vi "CRYCalc Pp value.vi"(0 "Data values in":T1 {"Z data" items=["dB", "Lin"]; "X data" items=["dB", "Lin"]; "Y data" items=["dB", "Lin"]; "Z dB ref" format="%.1f"; "Z axis" items=["Log", "Lin"]; "X dB ref" format="%.1f"; "X axis" items=["Log", "Lin"]; "Y axis" items=["Log", "Lin"]; "Y dB ref" format="%.1f"; "Curve"."z" format="%.2f"; "Curve"."y" format="%.2f"; "Curve"."x" format="%.2f"}, 1 "Step Setup VI No":i32, 5 "USL":dbl, 9 "LSL":dbl, 11 "Statistic Run Number":i32, 12 "Mode xyz":u16, 13 "Work in":u16) -> (4 "Pp value Out":T1 {"Z data" items=["dB", "Lin"]; "X data" items=["dB", "Lin"]; "Y data" items=["dB", "Lin"]; "Z dB ref" format="%.1f"; "Z axis" items=["Log", "Lin"]; "X dB ref" format="%.1f"; "X axis" items=["Log", "Lin"]; "Y axis" items=["Log", "Lin"]; "Y dB ref" format="%.1f"; "Curve"."z" format="%.2f"; "Curve"."y" format="%.2f"; "Curve"."x" format="%.2f"}, 6 "Mean Out":T1 {"Z data" items=["dB", "Lin"]; "X data" items=["dB", "Lin"]; "Y data" items=["dB", "Lin"]; "Z dB ref" format="%.1f"; "Z axis" items=["Log", "Lin"]; "X dB ref" format="%.1f"; "X axis" items=["Log", "Lin"]; "Y axis" items=["Log", "Lin"]; "Y dB ref" format="%.1f"; "Curve"."z" format="%.2f"; "Curve"."y" format="%.2f"; "Curve"."x" format="%.2f"}, 10 "Absolute StanDev Out":T1 {"Z data" items=["dB", "Lin"]; "X data" items=["dB", "Lin"]; "Y data" items=["dB", "Lin"]; "Z dB ref" format="%.1f"; "Z axis" items=["Log", "Lin"]; "X dB ref" format="%.1f"; "X axis" items=["Log", "Lin"]; "Y axis" items=["Log", "Lin"]; "Y dB ref" format="%.1f"; "Curve"."z" format="%.2f"; "Curve"."y" format="%.2f"; "Curve"."x" format="%.2f"})   [LabVIEW 2013]
uses:
  Typedef Control/CRYData Cluster Array.ctl
  Typedef Control/CRYData Cluster.ctl
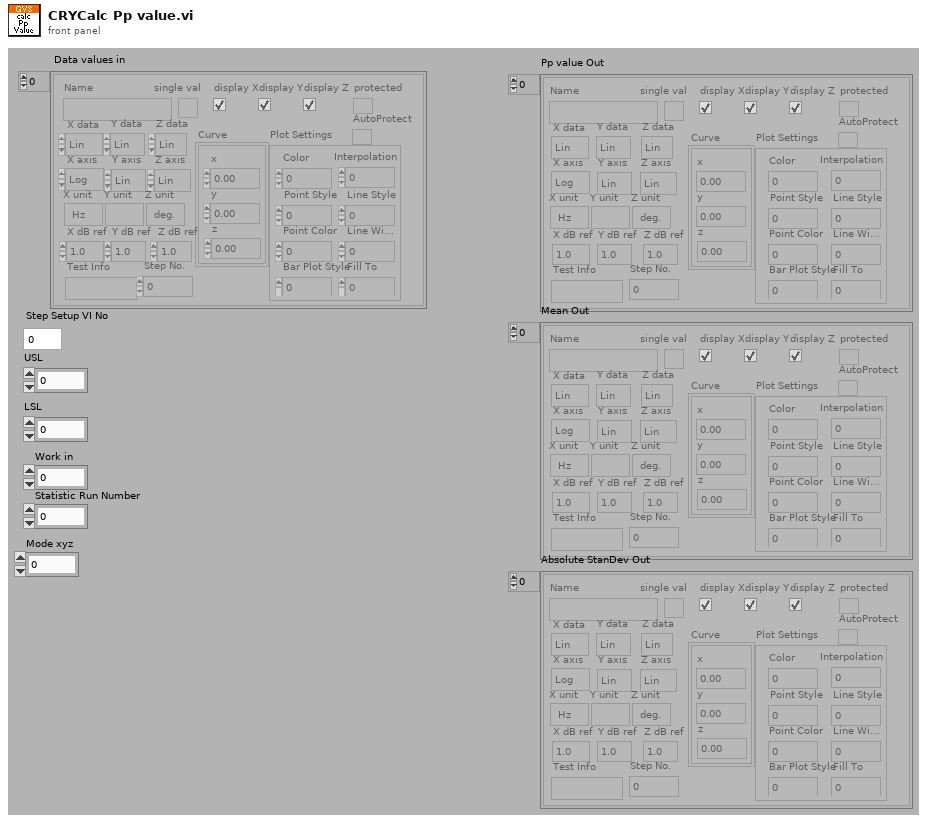
[diagram p1: front panel]
types:
  T1 = typedef "CRYData Cluster Array.ctl" = T2[]
  T2 = typedef "CRYData Cluster.ctl" = cluster{"Name":string, "Curve":cluster{"x":dbl, "y":dbl, "z":dbl}[], "X data":u16, "Y data":u16, "Z data":u16, "X axis":u16, "Y axis":u16, "Z axis":u16, "X unit":string, "Y unit":string, "Z unit":string, "X dB ref":dbl, "Y dB ref":dbl, "Z dB ref":dbl, "single val":bool, "protected":bool, "display X":bool, "display Y":bool, "display Z":bool, "Test Info":string, "Step No.":i32, "Plot Settings":cluster{"Color":u32, "Interpolation":u8, "Point Style":u8, "Line Style":u8, "Point Color":u32, "Line Width":u8, "Bar Plot Style":u8, "Fill To":i16}, "AutoProtect":bool}
  T3 = enum32{"English", "Chinese", "Korean", "Japanese", "Russian", "Chinese traditional"}
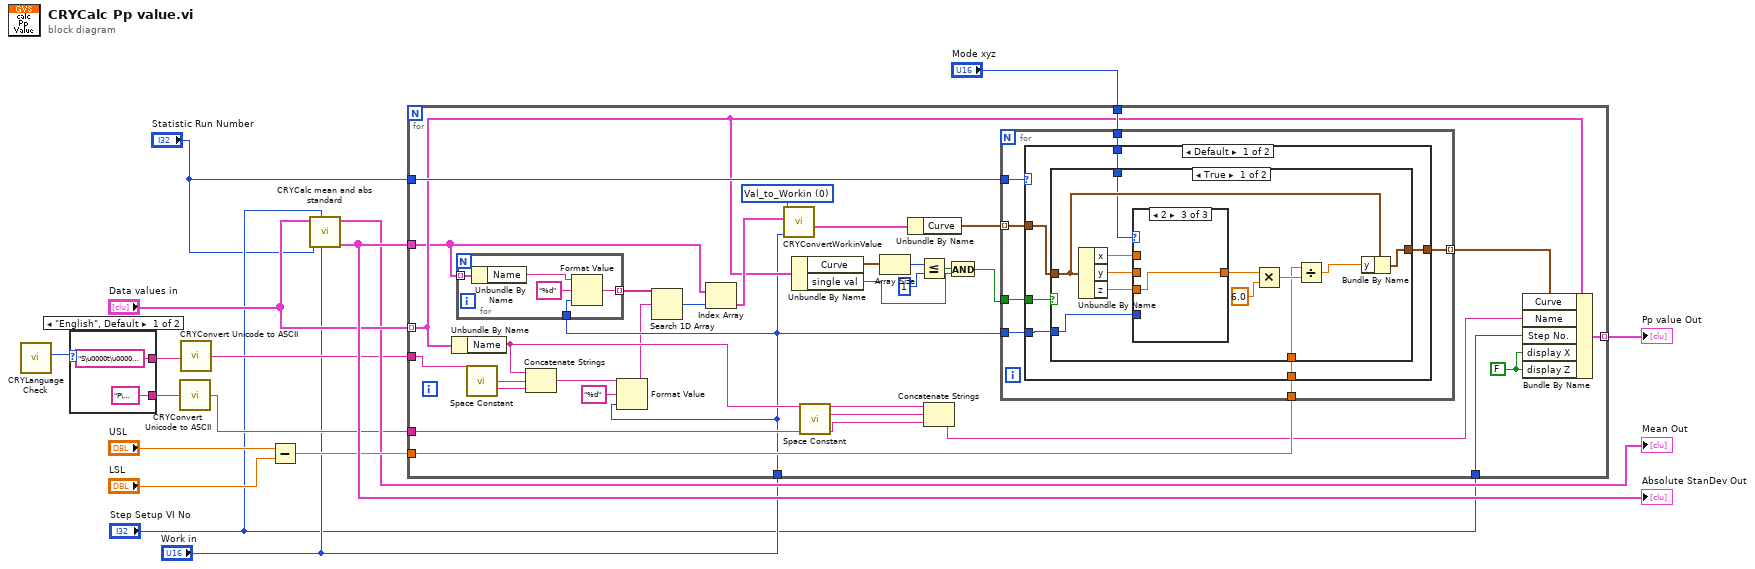
[diagram p0: block diagram]
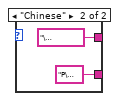
[diagram p2: hidden frame]
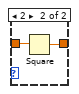
[diagram p5: hidden frame]
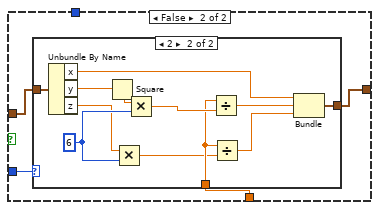
[diagram p6: hidden frame]
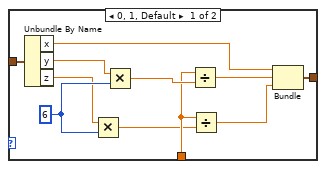
[diagram p7: hidden frame]
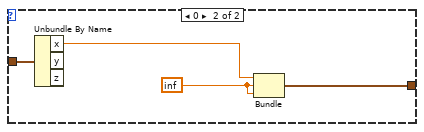
[diagram p8: hidden frame]
diagram:
  n1 = call "CRYLanguage Check.vi"() -> ("Language"=w9:T3)  [unwired: 10 in, 1 out]
  n2 = case shown="\"English\", Default" w9 {
    tunnel: ["S\u0000t\u0000d\u0000 \u0000D\u0000e\u0000v\u0000" ("format string") "\u0007hÆQî]" ("format string")] -> w8
    tunnel: ["P\u0000p\u0000" ("format string") "P\u0000p\u0000" ("format string")] -> w7
    frame "English", Default {
    }
    frame "Chinese" {
    }
  }
  n3 = call "CRYConvert Unicode to ASCII.vi"("Unicode"=w7) -> ("ASCII"=w5:string)  [unwired: 4 in]
  n4 = call "CRYConvert Unicode to ASCII.vi"("Unicode"=w8) -> ("ASCII"=w6:string)  [unwired: 4 in]
  n5 = Subtract(x="USL", y="LSL") -> (x-y=w12:dbl)
  n6 = call "CRYCalc mean and abs standard.vi"("Work in"="Work in", "Step Setup VI No"="Step Setup VI No", "Statistic Run Number"="Statistic Run Number", "Data in"="Data values in") -> ("Absolute StanDev Out"=w14:T1, "Mean Out"=→"Mean Out":T1)  [unwired: 5 in, 1 out]
  "Absolute StanDev Out" <- w14
  n7 = for {
    tunnel: w14 -> [w26]
    tunnel: "Data values in" -> [w27] mode=indexing
    tunnel: w12 -> [w47]
    tunnel: [w37] -> w11 mode=indexing
    tunnel: "Step Setup VI No" -> [w43]
    tunnel: w6 -> [w42]
    tunnel: w5 -> [w41]
    tunnel: "Work in" -> [w22]
    tunnel: "Statistic Run Number" -> [w36]
    tunnel: "Mode xyz" -> [w35]
    w34 = FALSE ("display X")
    w38 = u16 0 items=["Val_to_Workin", "Workin_to_ Val"] ("Type")
    n8 = Unbundle By Name(w27) -> ("Name"=w48:string)
    n9 = for {
      tunnel: w26 -> [w56] mode=indexing
      tunnel: w22 -> [w53]
      tunnel: [w52] -> w25 mode=indexing
      n10 = Unbundle By Name(w56) -> ("Name"=w54:string)
      n11 = Format Value(string ("")=w54, format string="%d", value (0)=w53) -> (output string=w52:string)
    }
    n12 = call <vilib>:"Space Constant.vi"() -> ("String"=w51:string)
    n13 = Concatenate Strings(w48, w51, w42) -> (w23:string)
    n14 = Format Value(string ("")=w23, format string="%d", value (0)=w22) -> (output string=w21:string)
    n15 = Search 1D Array(1D array=w25, element=w21) -> (index of element=w50:i32)  [unwired: 1 in]
    n16 = Index Array(array=w26, index=w50) -> (element=w40:T2)
    n17 = call "CRYConvertWorkinValue.vi"("Work in"=w22, "In"=w40, "Type"=w38) -> ("Out"=w39:T2)  [unwired: 8 in]
    n18 = Unbundle By Name(w27) -> ("Curve"=w33:cluster{"x":dbl, "y":dbl, "z":dbl}[], "single val"=w29:bool)
    n19 = call <vilib>:"Space Constant.vi"() -> ("String"=w49:string)
    n20 = Array Size(array=w33) -> (size(s)=w32:i32)
    n21 = Unbundle By Name(w39) -> ("Curve"=w44:cluster{"x":dbl, "y":dbl, "z":dbl}[])
    n22 = Less Or Equal?(x=w32, y=1) -> (x <= y?=w30:bool)
    n23 = Concatenate Strings(w48, w49, w41) -> (w46:string)
    n24 = And(x=w30, y=w29) -> (x .and. y?=w28:bool)
    n25 = for {
      tunnel: w44 -> [w63] mode=indexing
      tunnel: w47 -> [w62]
      tunnel: [w61] -> w45 mode=indexing
      tunnel: w22 -> [w60]
      tunnel: w36 -> [w59]
      tunnel: w28 -> [w58]
      tunnel: w35 -> [w57]
      n26 = case shown="Default" w59 {
        tunnel: w63 -> [w69 w120]
        tunnel: w62 -> [w68 _]
        tunnel: [w67 w119] -> w61
        tunnel: w60 -> [w66 _]
        tunnel: w58 -> [w65 _]
        tunnel: w57 -> [w64 _]
        frame Default {
          n27 = case shown="True" w65 {
            tunnel: w69 -> [w81 w93]
            tunnel: w68 -> [w73 w92]
            tunnel: [w80 w91] -> w67
            tunnel: w66 -> [w76 w90]
            tunnel: w64 -> [w70 _]
            frame True {
              n28 = Unbundle By Name(w81) -> ("x"=w75:dbl, "y"=w79:dbl, "z"=w74:dbl)
              n29 = case shown="2" w70 {
                tunnel: w79 -> [_ w85 _]
                tunnel: [w82 w84 w89] -> w78
                tunnel: w76 -> [_ w83 _]
                tunnel: w75 -> [w82 _ _]
                tunnel: w74 -> [_ _ w89]
                frame 0, Default {
                }
                frame 1 {
                  n30 = case shown="0, 1, Default" w83 {
                    tunnel: w85 -> [w86 w88]
                    tunnel: [w86 w87] -> w84
                    frame 0, 1, Default {
                    }
                    frame 2 {
                      n31 = Square(x=w88) -> (x^2=w87:dbl)
                    }
                  }
                }
                frame 2 {
                }
              }
              n32 = Multiply(x=w78, y=6.0) -> (x*y=w77:dbl)
              n33 = Divide(x=w73, y=w77) -> (x/y=w71:dbl)
              n34 = Bundle By Name(cluster=w81, "y"=w71) -> (w80:cluster{"x":dbl, "y":dbl, "z":dbl})
            }
            frame False {
              n35 = case shown="2" w90 {
                tunnel: w93 -> [w104 w116]
                tunnel: w92 -> [w101 w113]
                tunnel: [w96 w107] -> w91
                frame 0, 1, Default {
                  w103 = 6 ("standard deviation")
                  n36 = Unbundle By Name(w104) -> ("x"=w98:dbl, "y"=w95:dbl, "z"=w94:dbl)
                  n37 = Multiply(x=w94, y=w103) -> (x*y=w100:dbl)
                  n38 = Multiply(x=w95, y=w103) -> (x*y=w102:dbl)
                  n39 = Divide(x=w101, y=w102) -> (x/y=w99:dbl)
                  n40 = Divide(x=w101, y=w100) -> (x/y=w97:dbl)
                  n41 = Bundle("x"=w98, w99, w97) -> (w96:cluster{"x":dbl, dbl, dbl})  [unwired: 1 in]
                }
                frame 2 {
                  w115 = 6 ("standard deviation")
                  n42 = Unbundle By Name(w116) -> ("x"=w109:dbl, "y"=w111:dbl, "z"=w105:dbl)
                  n43 = Square(x=w111) -> (x^2=w106:dbl)
                  n44 = Multiply(x=w105, y=w115) -> (x*y=w112:dbl)
                  n45 = Multiply(x=w106, y=w115) -> (x*y=w114:dbl)
                  n46 = Divide(x=w113, y=w114) -> (x/y=w110:dbl)
                  n47 = Divide(x=w113, y=w112) -> (x/y=w108:dbl)
                  n48 = Bundle("x"=w109, w110, w108) -> (w107:cluster{"x":dbl, dbl, dbl})  [unwired: 1 in]
                }
              }
            }
          }
        }
        frame 0 {
          w117 = inf
          n49 = Unbundle By Name(w120) -> ("x"=w118:dbl)  [unwired: 2 out]
          n50 = Bundle("x"=w118, w117, w117) -> (w119:cluster{"x":dbl, dbl, dbl})  [unwired: 1 in]
        }
      }
    }
    n51 = Bundle By Name(cluster=w27, "Curve"=w45, "Name"=w46, "Step No."=w43, "display X"=w34, "display Z"=w34) -> (w37:T2)
  }
  "Pp value Out" <- w11
